vi "initialize user event if needed.vi"(11 "User Event in":T1) -> (3 "User Event out":T1)   [LabVIEW 2013, in "tag bus processing plugin editor node.lvclass"]
uses:
  tag bus processing plugin editor node.lvclass
  <vilib>/CEF_TreeControl/Node/UserEventRef.ctl
  <vilib>/CEF_TreeControl/Controls/EventCluster.ctl
  <vilib>/CEF_TreeControl/NISE_CEF_TreeControl.lvlib
  <vilib>/CEF_TreeControl/Node/NISE_CEF_Node.lvclass
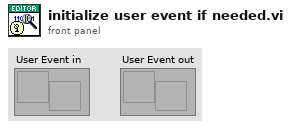
[diagram p1: front panel]
types:
  T1 = typedef "NISE_CEF_Node.lvclass/UserEventRef.ctl" = refnum<user-event>
  T2 = typedef "NISE_CEF_TreeControl.lvlib/EventCluster.ctl" = cluster{"command":string, "data":string}
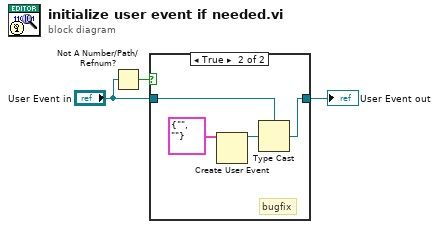
[diagram p0: block diagram]
diagram:
  n1 = Not A Number/Path/Refnum?(number/path/refnum="User Event in") -> (NaN/Path/Refnum?=w3:bool)
  n2 = case shown="True" w3 {
    tunnel: "User Event in" -> [w4 w5]
    tunnel: [w4 w6] -> w1
    frame False {
    }
    frame True {
      # "bugfix"
      n3 = Create User Event(user event datatype=T2 {"command"="", "data"=""} ("event data")) -> (user event=w7:refnum<user-event>)  [unwired: 1 in, 1 out]
      n4 = Type Cast(type=w5, x=w7) -> (*(type *) &x=w6:T1)
    }
  }
  "User Event out" <- w1
